vi "SerialPortMachine.vi"(2 "IRQ Number":u8, 3 "Port":refnum<k21>, 4 "FIFOout":refnum<k21>, 5 "Instructions":refnum<k21>) -> ()   [LabVIEW 2018]
uses:
  <vilib>/LabVIEW Targets/FPGA/cRIO/shared/nicrio_ModuleControls/nicrio_cRIO-9871_DataBitsEnum.ctl
  <vilib>/rvi/Emulation/niFpgaGetClockAttributes.vi
  <vilib>/rvi/Emulation/niFpgaSctlEmulationGetInTimedLoop.vi
  <vilib>/rvi/Emulation/niFpgaEmulationReportErrorSimple.vi
  <vilib>/rvi/DataTransferAndStorage/Container/Common/niFpgaContainerGetUniqueNameForEmu.vi
  <vilib>/rvi/DataTransferAndStorage/Container/Common/niFpgaContainerSetEmuInfo.vi
  <vilib>/rvi/eio/common/nirviEmuReportErrorAndStop.vi
  <vilib>/rvi/DataTransferAndStorage/Container/Common/niFpgaContainerExecOnDevCompGetState.vi
  <vilib>/rvi/Emulation/niFpgaEmulationIsFPGAContextNoSignature.vi
  <vilib>/rvi/errors/niFpgaSetErrorForExecOnDevCompSimple.vi
  <vilib>/rvi/FIFO/Fifo_Resource/nirvififoEmulationSetSize.vi
  <vilib>/rvi/FIFO/Fifo_Resource/nirviFifoEmulationQueueMgr.vi
  <instcachedir>/0/nirviFifoEmulationQueueMgr_E5CAEC123FF24DC58D834DCA3CDAA9B5.lvgen/nirviFifoEmulationQueueMgr_E5CAEC123FF24DC58D834DCA3CDAA9B5_001.vi
  <vilib>/rvi/FIFO/Fifo_Resource/nirvififoEmulationDetermineInputValidOut.vi
  <vilib>/rvi/FIFO/Fifo_Resource/nirvififoEmulationCreateLock.vi
  <vilib>/rvi/Emulation/niFpgaProcessEmulError.vi
  <vilib>/rvi/FIFO/Fifo_Resource/nirvififoEmulationObtainLock.vi
  <vilib>/rvi/FIFO/Fifo_Resource/nirvififoEmulationReleaseLock.vi
  <vilib>/rvi/occurrence/nirviWaitOnOccurrenceBase.vi
  <vilib>/rvi/errors/nirviReportUnexpectedCaseInternalError.vi
  <vilib>/rvi/errors/nirviReportUnexpectedCaseInternalError (U32).vi
  <vilib>/Utility/error.llb/Clear Errors.vi
  <vilib>/rvi/interface/RandomDataEmulation/niFpgaRandomDataHandleErrors.vi
  <vilib>/rvi/eio/common/nirviEmuTemplatePropertyGet_noerrors.vi
  <vilib>/rvi/Memory/Memory_Emulation/niFpgaMemoryEmulationCacheClearOnFirstRun.vi
  <vilib>/rvi/Memory/Memory_Emulation/nirvimemoryEmulationManagerCache_MakeExclusive.vi
  <vilib>/rvi/Memory/Memory_Emulation/niFpgaMemoryEmulationValidateCache.vi
  <vilib>/rvi/Memory/Memory_Emulation/nirvimemoryEmulationManagerCache_InsertValue.vi
  <vilib>/rvi/Memory/Memory_Emulation/nirvimemoryEmulationManagerCache_ReleaseExclusive.vi
  <vilib>/rvi/Memory/Memory_Emulation/nirvimemoryEmulationManagerCache_GetValue.vi
  <vilib>/rvi/Memory/Memory_Emulation/nirvimemoryEmulationManagerCache_SetValue.vi
  <vilib>/rvi/eio/common/nirviEmuTemplateMethod_errors.vi
  <vilib>/rvi/Emulation/niFpgaCriticalErrorInLSC.vi
  <vilib>/rvi/LocalResourceManager/LocalResourceManager.xnode
  <vilib>/rvi/DataTransferAndStorage/Container/XNode/niFpgaContainer.xnode
  <vilib>/rvi/FIFO/Fifo_Resource/niFpgaFifoEmulationRefIn.vi
  <vilib>/eio/EIOPropertyNode/EIOPropertyNode.xnode
  <vilib>/LabVIEW Targets/FPGA/cRIO/shared/nicrio_ModuleControls/nicrio_cRIO-9871_BaudRatePrescalerEnum.ctl
  <vilib>/LabVIEW Targets/FPGA/cRIO/shared/nicrio_ModuleControls/nicrio_cRIO-9871_FlowControlEnum.ctl
  <vilib>/LabVIEW Targets/FPGA/cRIO/shared/nicrio_ModuleControls/nicrio_cRIO-9871_StopBitsEnum.ctl
  <vilib>/LabVIEW Targets/FPGA/cRIO/shared/nicrio_ModuleControls/nicrio_cRIO-9871_ParityEnum.ctl
  <vilib>/rvi/DataTransferAndStorage/Register/Emulation/niFpgaRegisterEmulationRefIn.vi
  <vilib>/eio/EIOMethodNode/EIOMethodNode.xnode
  <vilib>/rvi/eio/common/nirviEmuTemplatePropertyGet_errors.vi
  <vilib>/rvi/eio/common/nirviEmuTemplatePropertySet_errors.vi
  <vilib>/rvi/eio/common/nirviEmuTemplatePropertySet_noerrors.vi
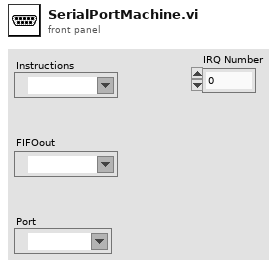
[diagram p1: front panel]
types:
  T1 = typedef "nicrio_cRIO-9871_DataBitsEnum.ctl" = enum8{"5", "6", "7", "8"}
  T2 = typedef "nicrio_cRIO-9871_BaudRatePrescalerEnum.ctl" = enum8{"1", "4"}
  T3 = typedef "nicrio_cRIO-9871_FlowControlEnum.ctl" = enum8{"None", "Software (XON / XOFF)", "Hardware (RTS / CTS)"}
  T4 = typedef "nicrio_cRIO-9871_StopBitsEnum.ctl" = enum8{"1", "1.5", "2"}
  T5 = typedef "nicrio_cRIO-9871_ParityEnum.ctl" = enum8{"None", "Odd", "Even", "Mark", "Space"}
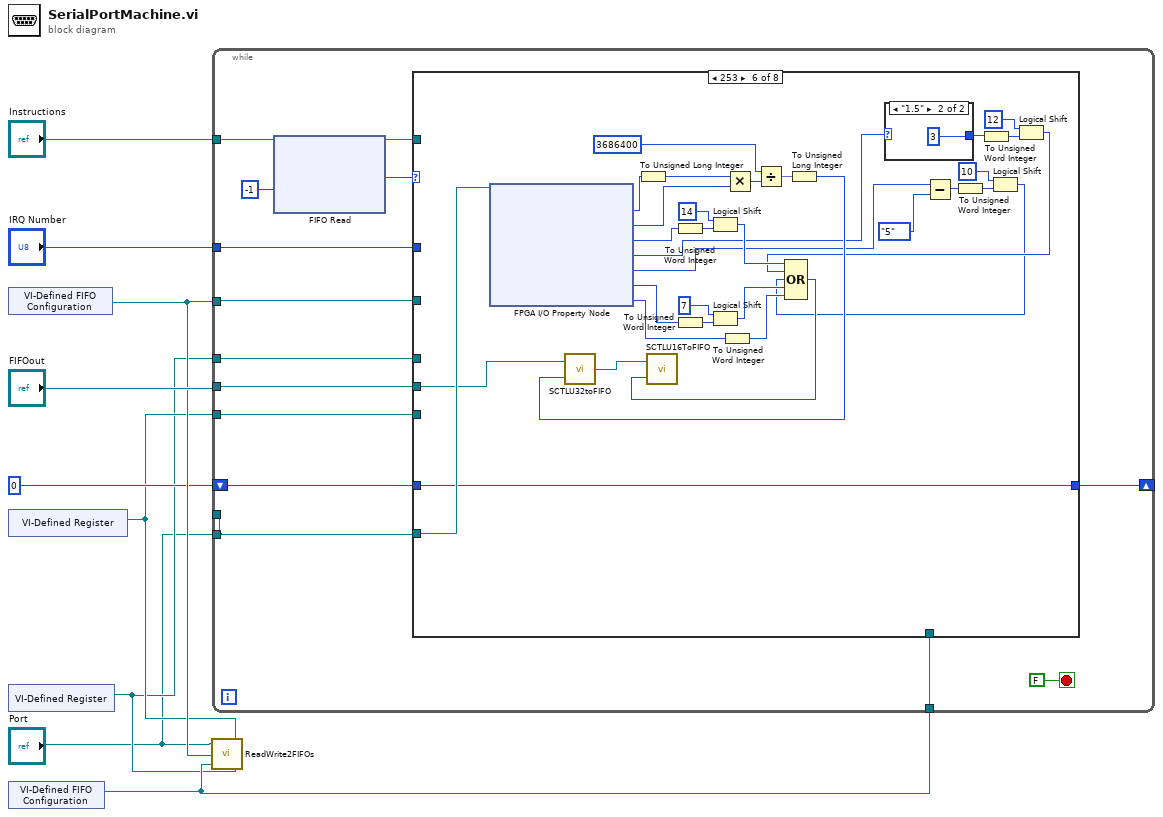
[diagram p0: block diagram]
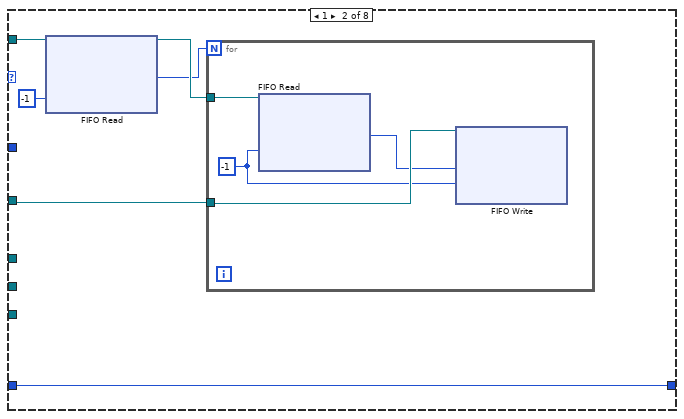
[diagram p3: hidden frame]
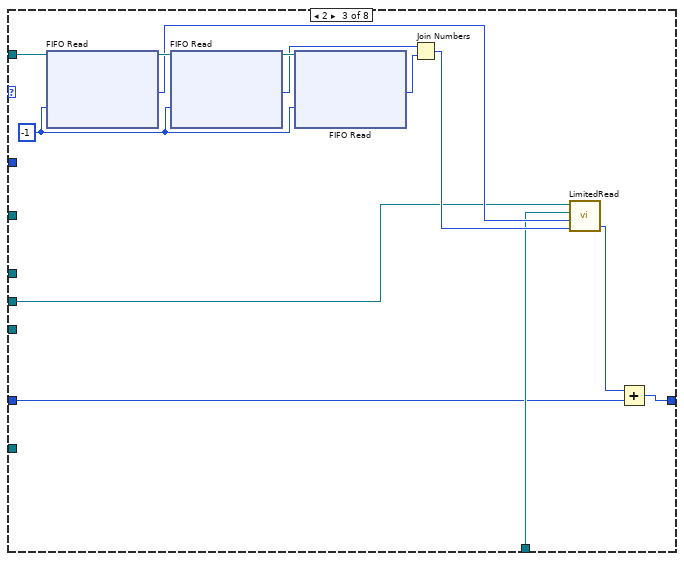
[diagram p4: hidden frame]
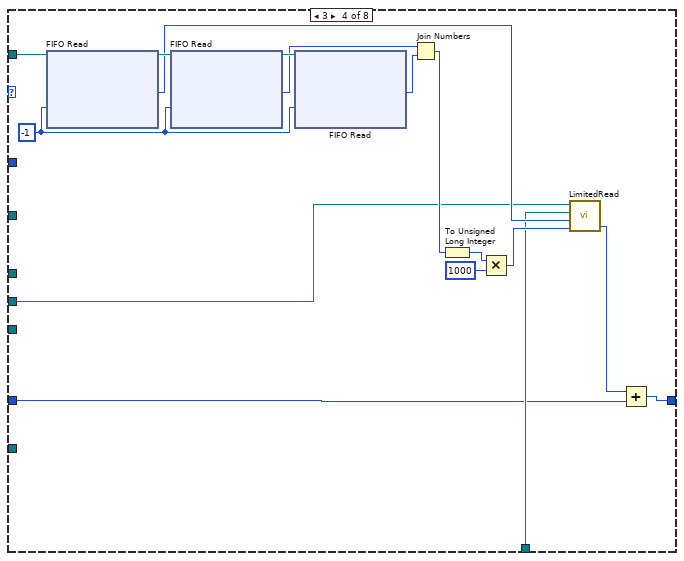
[diagram p5: hidden frame]
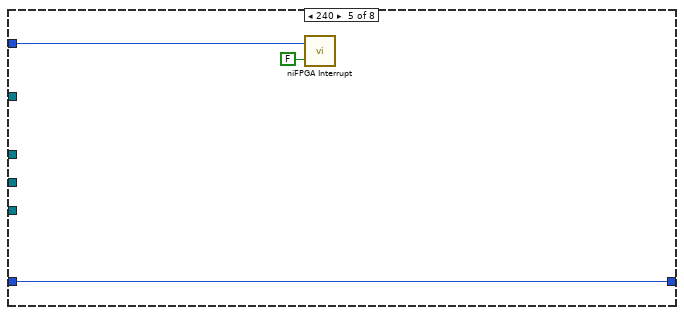
[diagram p6: hidden frame]
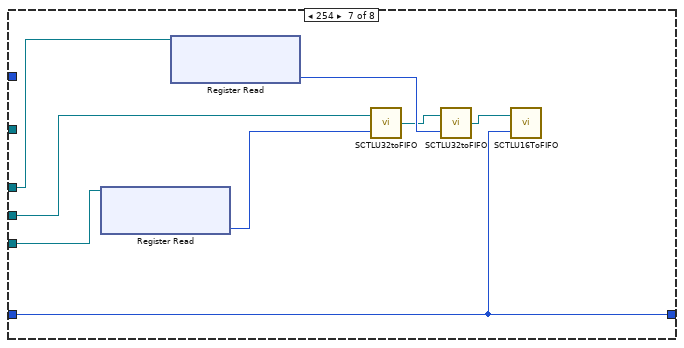
[diagram p8: hidden frame]
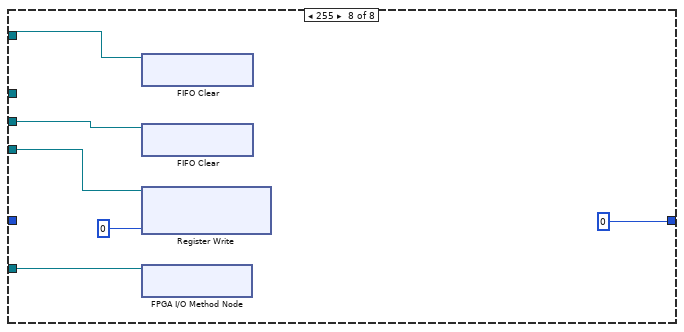
[diagram p9: hidden frame]
diagram:
  n1 = xnode "VI-Defined FIFO Configuration"() -> ("FIFO Out"=w7:refnum<k21>)
  n2 = xnode "VI-Defined Register"() -> ("Register Out"=w4:refnum<k21>)
  n3 = xnode "VI-Defined Register"() -> ("Register Out"=w3:refnum<k21>)
  n4 = xnode "VI-Defined FIFO Configuration"() -> ("FIFO Out"=w5:refnum<k21>)
  n5 = call "ReadWrite2FIFOs.vi"("ReadBytes"=w3, "WrittenBytes"=w4, "Reads"=w5, "Writes"=w7, "Port"="Port") -> ()
  n6 = while {
    tunnel: "Instructions" -> [w20]
    tunnel: w7 -> [w15]
    tunnel: w5 -> [w18]
    shift-right: [w16] -> _
    shift-left: u16 0 -> [w17]
    tunnel: "FIFOout" -> [w14]
    tunnel: w4 -> [w13]
    tunnel: w3 -> [w12]
    tunnel: "Port" -> [w10]
    tunnel: "IRQ Number" -> [w11]
    tunnel: [w10] -> _
    stop <- FALSE stop-if-true
    n7 = xnode ("FIFO Read")("Timeout"=-1, "FIFO In"=w20) -> ("Element"=w19:u8, "FIFO Out"=w21:refnum<k21>)  [unwired: 1 out]
    n8 = case shown="253" w19 {
      tunnel: w21 -> [_ w29 w47 w63 _ _ _ _]
      tunnel: w15 -> [_ w30 _ _ _ _ _ w114]
      tunnel: w18 -> [_ _ w39 w52 _ _ _ _]
      tunnel: w17 -> [w24 w25 w37 w51 w66 w93 w109 _]
      tunnel: [w24 w25 w38 w50 w66 w93 w109 u8 0 ("f")] -> w16
      tunnel: w14 -> [_ _ w36 w49 _ w81 w108 w113]
      tunnel: w13 -> [_ _ _ _ _ _ w107 w112]
      tunnel: w12 -> [_ _ _ _ _ _ w105 _]
      tunnel: w10 -> [_ _ _ _ _ w99 _ w110]
      tunnel: w11 -> [_ _ _ _ w64 _ _ _]
      frame 0, Default {
      }
      frame 1 {
        n9 = xnode ("FIFO Read")("Timeout"=-1, "FIFO In"=w29) -> ("Element"=w26:u8, "FIFO Out"=w27:refnum<k21>)  [unwired: 1 out]
        n10 = for {
          N: w26 -> [_]
          tunnel: w30 -> [w34]
          tunnel: w27 -> [w31]
          w32 = -1 ("Timeout")
          n11 = xnode ("FIFO Read")("Timeout"=w32, "FIFO In"=w31) -> ("Element"=w33:u8)  [unwired: 2 out]
          n12 = xnode ("FIFO Write")("Element"=w33, "Timeout"=w32, "FIFO In"=w34) -> ()  [unwired: 2 out]
        }
      }
      frame 2 {
        w42 = -1 ("Timeout")
        n13 = xnode ("FIFO Read")("Timeout"=w42, "FIFO In"=w47) -> ("Element"=w41:u8, "FIFO Out"=w46:refnum<k21>)  [unwired: 1 out]
        n14 = xnode ("FIFO Read")("Timeout"=w42, "FIFO In"=w46) -> ("Element"=w44:u8, "FIFO Out"=w45:refnum<k21>)  [unwired: 1 out]
        n15 = xnode ("FIFO Read")("Timeout"=w42, "FIFO In"=w45) -> ("Element"=w43:u8)  [unwired: 2 out]
        n16 = Join Numbers(hi=w44, lo=w43) -> ((hi.lo)=w40:u16)
        n17 = call "LimitedRead.vi"("MaxTime"=w40, "MaxLength"=w41, "ReadFIFO"=w39, "OutFIFO"=w36) -> ("Timedout"=w35:u8)  [unwired: 1 in, 1 out]
        n18 = Add(x=w35, y=w37) -> (x+y=w38:u16)
      }
      frame 3 {
        w58 = -1 ("Timeout")
        n19 = xnode ("FIFO Read")("Timeout"=w58, "FIFO In"=w63) -> ("Element"=w57:u8, "FIFO Out"=w62:refnum<k21>)  [unwired: 1 out]
        n20 = xnode ("FIFO Read")("Timeout"=w58, "FIFO In"=w62) -> ("Element"=w60:u8, "FIFO Out"=w61:refnum<k21>)  [unwired: 1 out]
        n21 = xnode ("FIFO Read")("Timeout"=w58, "FIFO In"=w61) -> ("Element"=w59:u8)  [unwired: 2 out]
        n22 = Join Numbers(hi=w60, lo=w59) -> ((hi.lo)=w56:u16)
        n23 = To Unsigned Long Integer(number=w56) -> (unsigned 32bit integer=w54:u32)
        n24 = Multiply(x=w54, y=u32 1000) -> (x*y=w55:u32)
        n25 = call "LimitedRead.vi"("MaxTime"=w55, "MaxLength"=w57, "ReadFIFO"=w52, "OutFIFO"=w49) -> ("Timedout"=w48:u8)  [unwired: 1 in, 1 out]
        n26 = Add(x=w48, y=w51) -> (x+y=w50:u16)
      }
      frame 240 {
        n27 = call <vilib>:"niFPGA Interrupt.vi"("Wait Until Cleared (F)"=FALSE, "IRQ Number (0)"=w64) -> ()  [unwired: 1 in]
      }
      frame 253 {
        n28 = xnode "FPGA I/O Property Node"("FPGA I/O In"=w99) -> ("Baud Rate Divider"=w97:u16, "Baud Rate Prescaler"=w96:T2, "Flow Control"=w91:T3, "Stop Bits"=w79:T4, "Data Bits"=w72:T1, "Parity"=w90:T5, "Bytes at Port"=w88:u8)  [unwired: 1 out]
        n29 = To Unsigned Long Integer(number=w97) -> (unsigned 32bit integer=w83:u32)
        n30 = To Unsigned Word Integer(number=w91) -> (unsigned 16bit integer=w85:u16)
        n31 = To Unsigned Word Integer(number=w90) -> (unsigned 16bit integer=w84:u16)
        n32 = Logical Shift(y=i16 14, x=w85) -> (x << y=w89:u16)
        n33 = Logical Shift(y=i16 7, x=w84) -> (x << y=w73:u16)
        n34 = To Unsigned Word Integer(number=w88) -> (unsigned 16bit integer=w74:u16)
        n35 = Multiply(x=w83, y=w96) -> (x*y=w94:u32)
        n36 = Divide(x=u32 3686400, y=w94) -> (x/y=w95:fxp<+/-,16,16>)
        n37 = To Unsigned Long Integer(number=w95) -> (unsigned 32bit integer=w82:u32)
        n38 = call "SCTLU32toFIFO.vi"("Number"=w82, "FifoIn"=w81) -> ("FifoOUT"=w80:refnum<k21>)
        n39 = case shown="\"1.5\"" w79 {
          selector: w79 -> [w100 _]
          tunnel: [w100 i16 3] -> w76
          frame "1", Default {
          }
          frame "1.5" {
          }
        }
        n40 = Subtract(x=w72, y=nicrio_cRIO-9871_DataBitsEnum."5") -> (x-y=w68:u8)
        n41 = To Unsigned Word Integer(number=w68) -> (unsigned 16bit integer=w69:u16)
        n42 = To Unsigned Word Integer(number=w76) -> (unsigned 16bit integer=w77:u16)
        n43 = Logical Shift(y=i16 10, x=w69) -> (x << y=w67:u16)
        n44 = Logical Shift(y=i16 12, x=w77) -> (x << y=w75:u16)
        n45 = Compound Arithmetic op=OR(w89, w75, w67, w73, w74) -> (w87:u16)
        n46 = call "SCTLU16ToFIFO.vi"("Number"=w87, "FifoIn"=w80) -> ()  [unwired: 1 out]
      }
      frame 254 {
        n47 = xnode ("Register Read")("Register In"=w107) -> ("Data"=w106:u32)  [unwired: 1 out]
        n48 = xnode ("Register Read")("Register In"=w105) -> ("Data"=w104:u32)  [unwired: 1 out]
        n49 = call "SCTLU32toFIFO.vi"("Number"=w106, "FifoIn"=w108) -> ("FifoOUT"=w103:refnum<k21>)
        n50 = call "SCTLU32toFIFO.vi"("Number"=w104, "FifoIn"=w103) -> ("FifoOUT"=w102:refnum<k21>)
        n51 = call "SCTLU16ToFIFO.vi"("Number"=w109, "FifoIn"=w102) -> ()  [unwired: 1 out]
      }
      frame 255 {
        n52 = xnode ("FIFO Clear")("FIFO In"=w114) -> ()  [unwired: 1 out]
        n53 = xnode ("FIFO Clear")("FIFO In"=w113) -> ()  [unwired: 1 out]
        n54 = xnode ("Register Write")("Data"=u32 0, "Register In"=w112) -> ()  [unwired: 1 out]
        n55 = xnode "FPGA I/O Method Node"("FPGA I/O In"=w110) -> ()  [unwired: 1 out]
      }
    }
  }
